vi "LLB Pre-Build CHM Build.vi"(6 "Top Level/Always Included VIs":path[](array[path]), 7 "Main Destination Path":path, 9 "Target Name":string, 10 "Build Specification Name":string, 11 "Project Path":path) -> (0 "error out":errorcluster)   [LabVIEW 2018]
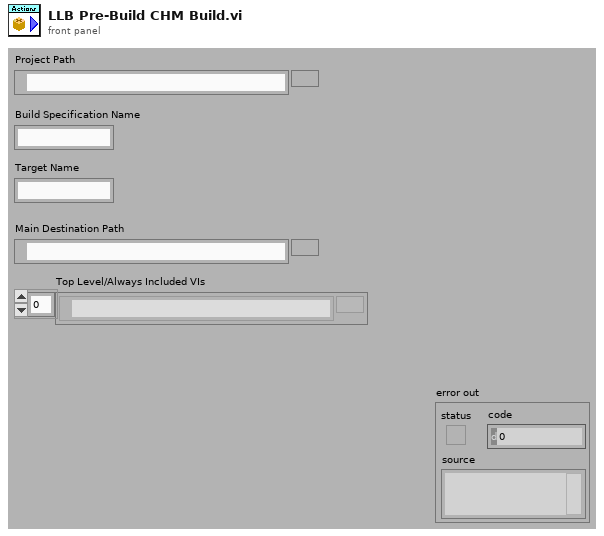
[diagram p1: front panel]
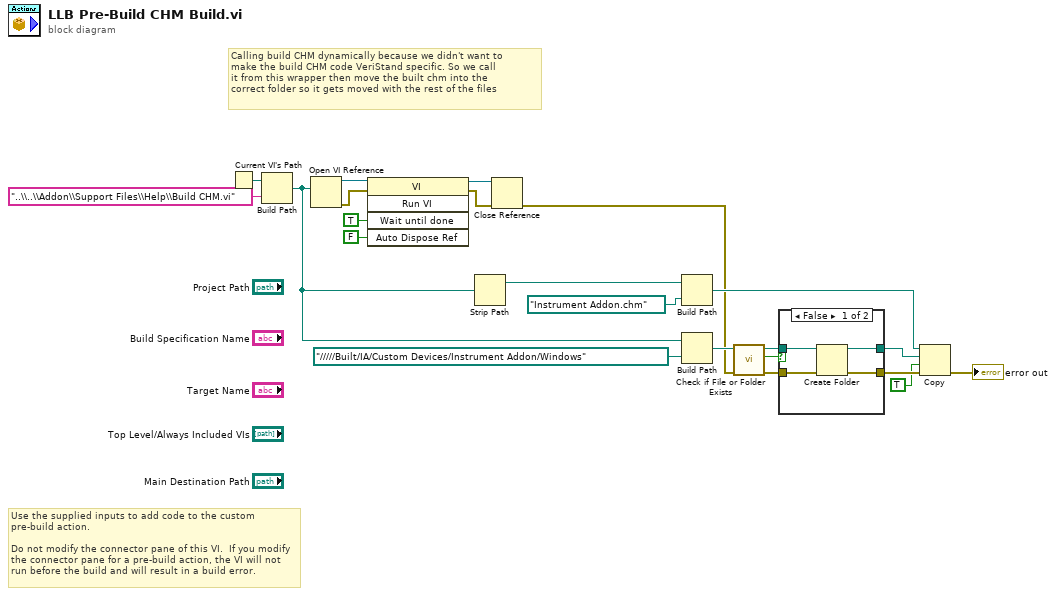
[diagram p0: block diagram]
diagram:
  # "Calling build CHM dynamically because we didn't want to \nmake the build CHM code VeriStand specific. So we call\nit from this wrapper then move the built chm into the\ncorrect folder so it gets moved with the rest of the files"
  # "Use the supplied inputs to add code to the custom pre-build action.\n\nDo not modify the connector pane of this VI.  If you modify the connector pane for a pre-build action, the VI will not run before the build and will result in a build error."
  n1 = Current VI's Path() -> (path=w22:path)
  n2 = Build Path(base path=w22, name or relative path="..\\..\\Addon\\Support Files\\Help\\Build CHM.vi") -> (appended path=w11:path)
  n3 = Open VI Reference(vi path=w11) -> (vi reference=w20:refnum<vi>, error out=w19:errorcluster)  [unwired: 5 in]
  n4 = invoke class="VI" method="Run VI"(reference=w20, error in=w19, "Wait until done"=TRUE ("Wait Until Done"), "Auto Dispose Ref"=FALSE ("Auto Dispose Reference")) -> (reference out=w16:refnum<vi>, error out=w15:errorcluster)  [unwired: 1 in, 3 out]
  n5 = Strip Path(path=w11) -> (stripped path=w14:path)  [unwired: 1 out]
  n6 = Close Reference(reference=w16, error in (no error)=w15) -> (error out=w1:errorcluster)
  n7 = Build Path(base path=w14, name or relative path=path "Instrument Addon.chm") -> (appended path=w5:path)
  n8 = Build Path(base path=w11, name or relative path=path "../../../../../Built/IA/Custom Devices/Instrument Addon/Windows") -> (appended path=w10:path)
  n9 = call <vilib>:"Check if File or Folder Exists.vi"("error in (no error)"=w1, "path"=w10) -> ("error out"=w7:errorcluster, "file or folder exists?"=w9:bool, "dup path"=w8:path)  [unwired: 7 in]
  n10 = case shown="False" w9 {
    tunnel: w8 -> [w25 w27]
    tunnel: w7 -> [w26 w28]
    tunnel: [w24 w27] -> w4
    tunnel: [w23 w28] -> w6
    frame False {
      n11 = Create Folder(path (use dialog)=w25, error in=w26) -> (created path=w24:path, error out=w23:errorcluster)  [unwired: 1 in, 1 out]
    }
    frame True {
    }
  }
  n12 = Copy(8:w6, 9:TRUE ("overwrite (F)"), 10:w4, 11:w5) -> (0:→"error out":errorcluster)  [unwired: 1 in, 2 out]
